vi "Allow UI_Read.vi"(8 "error in (no error)":errorcluster, 11 "Dependency Source in":refnum<class "Dependency Source.lvclass">) -> (0 "error out":errorcluster, 2 "Allow UI?":bool=TRUE, 3 "Dependency Source out":refnum<class "Dependency Source.lvclass">)   [LabVIEW 2019, in "Project.Dependencies Finder.lvlib" / "Dependency Source.lvclass"]
uses:
  Dependency Source.lvclass
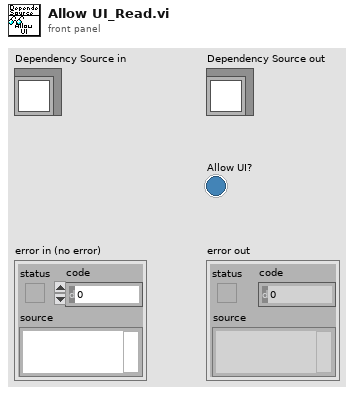
[diagram p1: front panel]
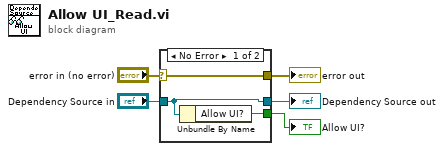
[diagram p0: block diagram]
diagram:
  n1 = case shown="No Error" "error in (no error)" {
    selector: "error in (no error)" -> [w8 w9]
    tunnel: [w8 w9] -> w4
    tunnel: [w7 w10] -> w2
    tunnel: "Dependency Source in" -> [w7 w10]
    tunnel: [w6 _] -> w1
    frame No Error {
      n2 = Unbundle By Name(w7) -> ("Allow UI?"=w6:bool)
    }
    frame Error {
    }
  }
  "error out" <- w4
  "Dependency Source out" <- w2
  "Allow UI?" <- w1
